vi "用户列表.vi"() -> ()   [LabVIEW 2016, in "Alarm interface.lvlib" / "wxpusher.lvlib"]
uses:
  wxpusher.lvlib
  <vilib>/Utility/miscctls.llb/LVPointTypeDef.ctl
panel:
  in  "关闭":bool
  in  "删除":bool
  in  "添加":bool
  in  "微信用户列表":i32(listbox)
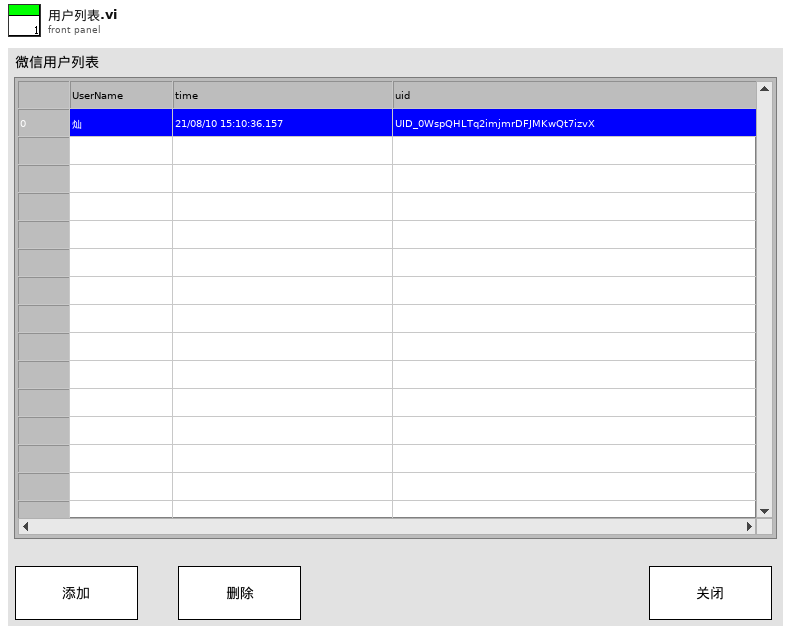
[diagram p1: front panel]
types:
  T1 = typedef "LVPointTypeDef.ctl" = cluster{"Horizontal":i16, "Vertical":i16}
  T2 = cluster{"action":string, "data":cluster{"appKey":string, "appName":string, "source":string, "time":u64, "uid":string, "userHeadImg":string, "userName":string, "extra":string}}[]
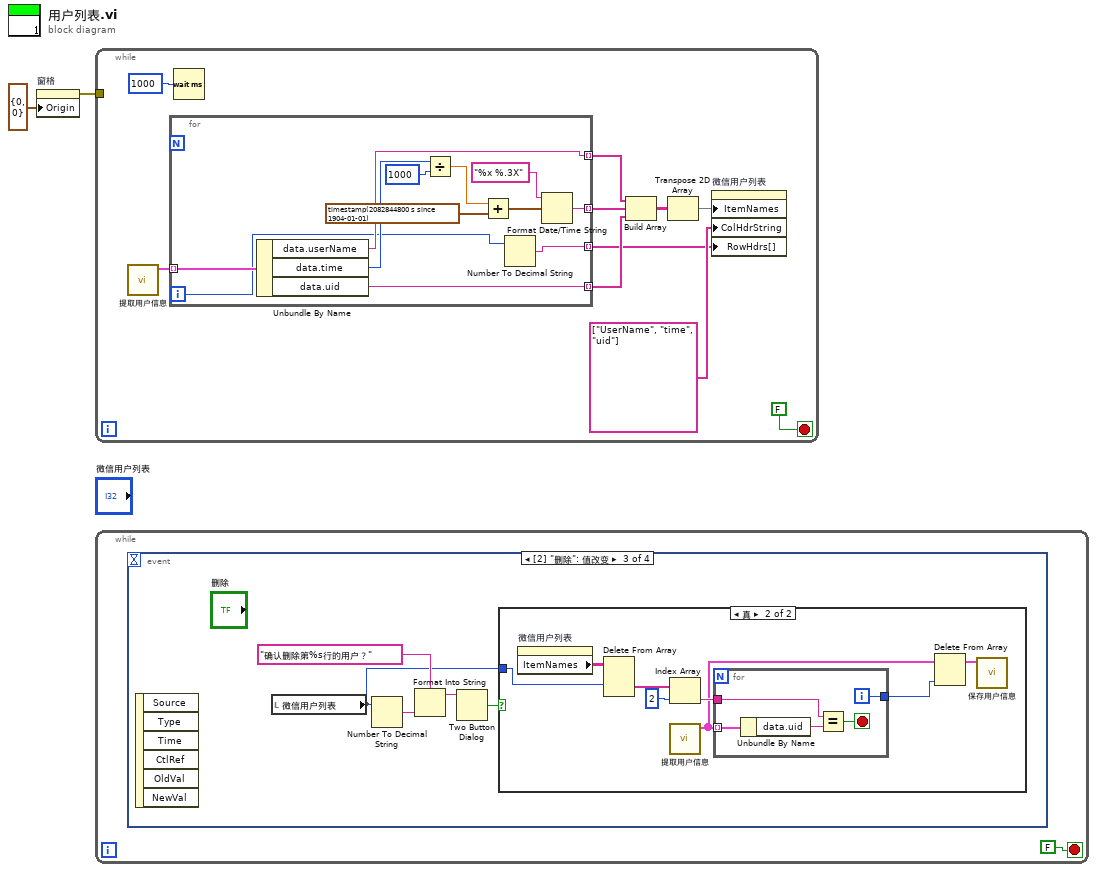
[diagram p0: block diagram]
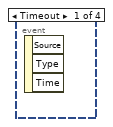
[diagram p2: hidden frame]
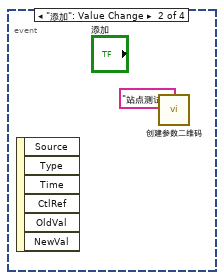
[diagram p3: hidden frame]
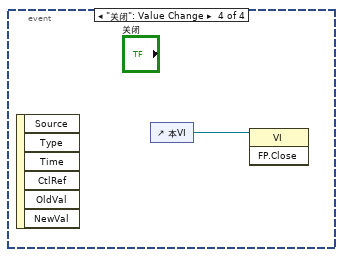
[diagram p5: hidden frame]
diagram:
  n1 = property on="窗格" class="Pane"("Origin"=T1 {"Horizontal"=0, "Vertical"=0} ("原点")) -> (error out=w1:errorcluster)  [unwired: 2 in, 1 out]
  n2 = while {
    tunnel: w1 -> [_]
    stop <- FALSE stop-if-true
    n3 = call "提取用户信息.vi"() -> ("用户信息"=w12:T2)  [unwired: 10 in, 1 out]
    n4 = for {
      tunnel: w12 -> [w24] mode=indexing
      tunnel: [w23] -> w11 mode=indexing
      tunnel: [w22] -> w9 mode=indexing
      tunnel: [w15] -> w10 mode=indexing
      tunnel: [w13] -> w3 mode=indexing
      i -> [w14]
      n5 = Unbundle By Name(w24) -> ("data.userName"=w23:string, "data.time"=w16:u64, "data.uid"=w22:string)
      n6 = Divide(x=w16, y=u64 1000) -> (x/y=w18:dbl)
      n7 = Add(x=w18, y=timestamp(2082844800 s since 1904-01-01)) -> (x+y=w20:timestamp)
      n8 = Number To Decimal String(number=w14) -> (decimal integer string=w13:string)  [unwired: 1 in]
      n9 = Format Date/Time String(time format string (%c)="%x %.3X" ("时间格式字符串(%c)"), seconds (now)=w20) -> (date/time string=w15:string)  [unwired: 1 in]
    }
    n10 = Wait (ms)(milliseconds to wait=u32 1000 ("等待时间（毫秒）")) -> ()  [unwired: 1 out]
    n11 = Build Array(w11, w10, w9) -> (w8:string[][])
    n12 = Transpose 2D Array(2D array=w8) -> (transposed array=w7:string[][])
    n13 = property on="微信用户列表" class="MCListbox (严格)"("ItemNames"=w7, "ColHdrString"=string[] ["UserName", "time", "uid"] ("列首字符串[]"), "RowHdrs[]"=w3) -> ()  [unwired: 2 in, 2 out]
  }
  n14 = while {
    stop <- FALSE stop-if-true
    n15 = event shown="[2] \"删除\": 值改变" {
      selector: _ -> [_ _ _ _]
      dyn-events: _ -> [_ _ _ _]
      timeout: _ -> [_ _ _ _]
      event Timeout {
        n16 = event-data() -> ()  [unwired: 1 in, 3 out]
      }
      event "添加": Value Change {
        n17 = event-data() -> ()  [unwired: 1 in, 6 out]
        n18 = call "创建参数二维码.vi"("站点"="站点测试") -> ()  [unwired: 11 in]
      }
      event "删除": Value Change {
        n19 = event-data() -> ()  [unwired: 1 in, 6 out]
        n20 = local read "微信用户列表"() -> (w30:i32)
        n21 = Number To Decimal String(number=w30) -> (decimal integer string=w29:string)  [unwired: 1 in]
        n22 = Format Into String(format string="确认删除第%s行的用户？" ("消息"), w29) -> (resulting string=w28:string)  [unwired: 2 in, 1 out]
        n23 = Two Button Dialog(message=w28) -> (T button?=w27:bool)  [unwired: 2 in]
        n24 = case shown="真" w27 {
          tunnel: w30 -> [_ w38]
          frame False {
          }
          frame True {
            n25 = property on="微信用户列表" class="MCListbox (严格)"() -> ("ItemNames"=w39:string[][])  [unwired: 2 in, 2 out]
            n26 = Delete From Array(array=w39, index (row)=w38) -> (deleted portion=w37:string[])  [unwired: 2 in, 1 out]
            n27 = Index Array(array=w37, index=2 ("索引")) -> (element=w35:string)
            n28 = call "提取用户信息.vi"() -> ("用户信息"=w34:T2)  [unwired: 10 in, 1 out]
            n29 = for {
              tunnel: w34 -> [w44] mode=indexing
              tunnel: w35 -> [w43]
              tunnel: [w40] -> w33
              i -> [w40]
              stop <- w41 stop-if-true
              n30 = Unbundle By Name(w44) -> ("data.uid"=w42:string)
              n31 = Equal?(x=w43, y=w42) -> (x = y?=w41:bool)
            }
            n32 = Delete From Array(array=w34, index=w33) -> (array with subset deleted=w32:T2)  [unwired: 1 in, 1 out]
            n33 = call "保存用户信息.vi"("用户信息"=w32) -> ()  [unwired: 10 in, 1 out]
          }
        }
      }
      event "关闭": Value Change {
        n34 = event-data() -> ()  [unwired: 1 in, 6 out]
        n35 = control-ref of="本VI"() -> (w45:refnum<vi>)
        n36 = invoke class="VI" method="FP.Close"(reference=w45) -> ()  [unwired: 2 in, 3 out]
      }
    }
  }
